vi "Data_PSD_267.vi"() -> ()   [LabVIEW 2020]
uses:
  <vilib>/Utility/error.llb/DialogType.ctl
  <vilib>/measure/maspectr.llb/Power Spectrum and PSD Export Mode.ctl
  <vilib>/Analysis/4window.llb/windowTd.ctl
  <vilib>/measure/maspectr.llb/FFT Power Spectrum and PSD for 1 Chan.vi
  <vilib>/Analysis/0measdsp.llb/Scaled Time Domain Window (DBL).vi
  <vilib>/sound2/lvsound2.llb/Sound File Info (path).vi
  <vilib>/sound2/lvsound2.llb/Sound File Read Open.vi
  <vilib>/sound2/lvsound2.llb/Sound File Read (DBL).vi
  <vilib>/Analysis/NI_AALPro.lvlib
  <vilib>/measure/NI_MAPro.lvlib
panel:
  in  "Stop":bool
  out "Data Cursor":T1
  in  "File Path":path
  out "Max Amplitude":dbl
  out "Frequency Peak":dbl
  out "Signal":waveform(dbl)(graph)
  out "PSD of Signal":cluster{"f0":dbl, "df":dbl, "magnitude":dbl[]}(graph)
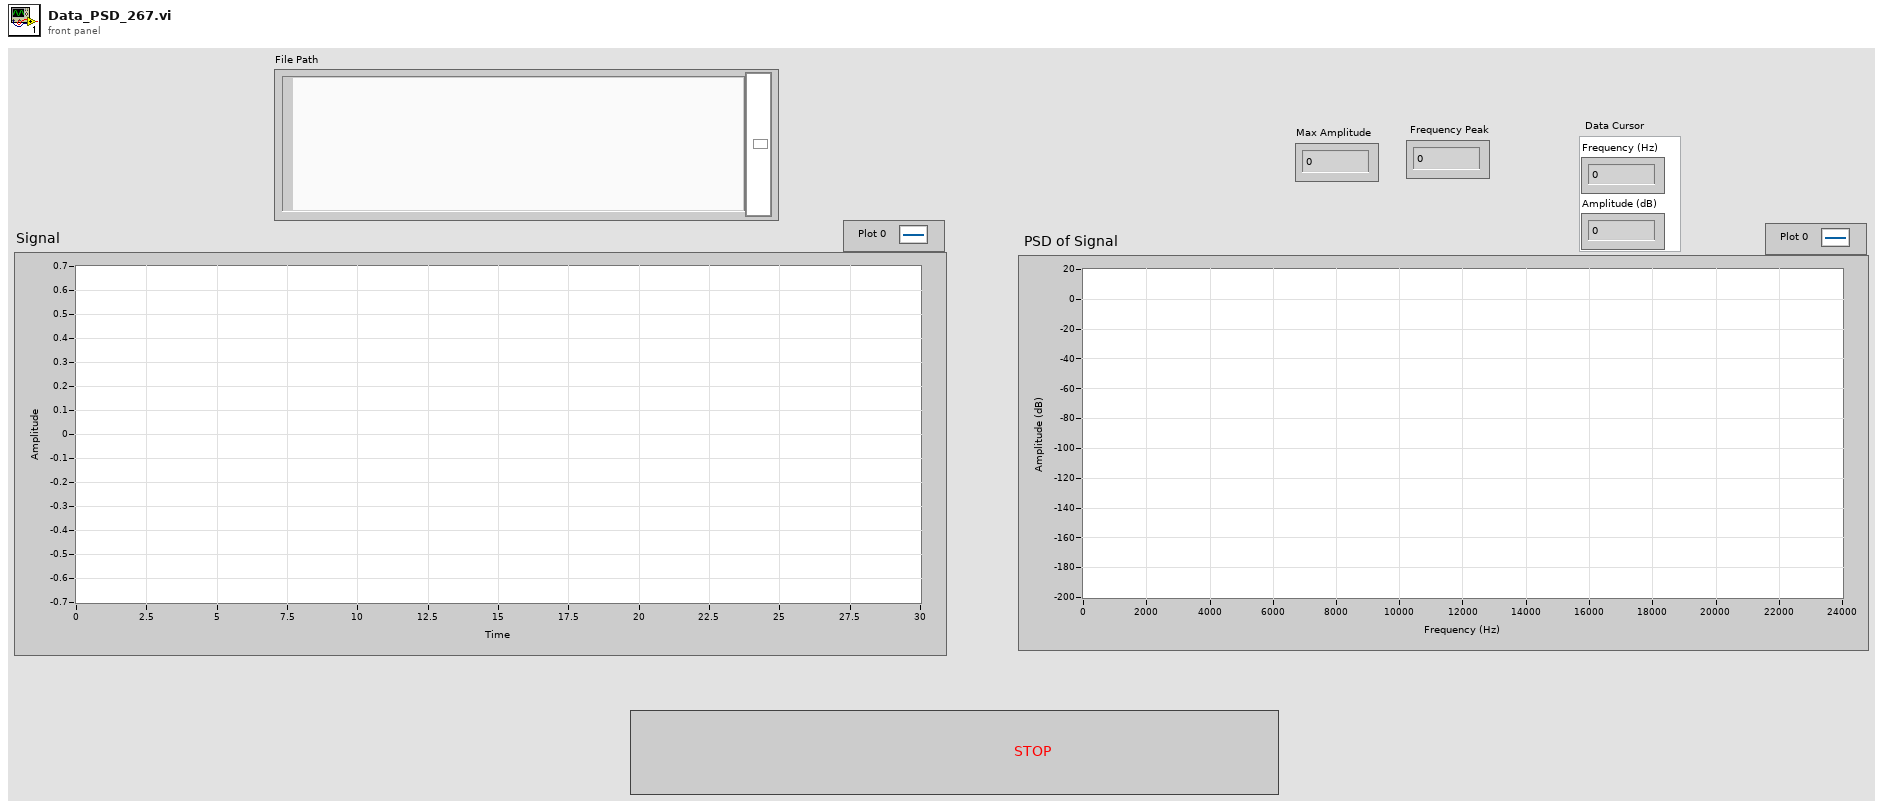
[diagram p1: front panel]
types:
  T1 = cluster{"Frequency (Hz)":dbl, "Amplitude (dB)":dbl}
  T2 = typedef "DialogType.ctl" = u16
  T3 = typedef "NI_AALPro.lvlib/windowTd.ctl" = u32
  T4 = typedef "NI_MAPro.lvlib/Power Spectrum and PSD Export Mode.ctl" = u16
  T5 = typedef "LVPointDoubleTypeDef.ctl" = cluster{"Cursor X":dbl, "Cursor Y":dbl}
  T6 = typedef "Sound File Refnum.ctl" = refnum<file>
  T7 = typedef "LVRangeTypeDef.ctl" = cluster{"Minimum":dbl, "Maximum":dbl, "Increment":dbl, "Minor Increment":dbl, "Start":dbl}
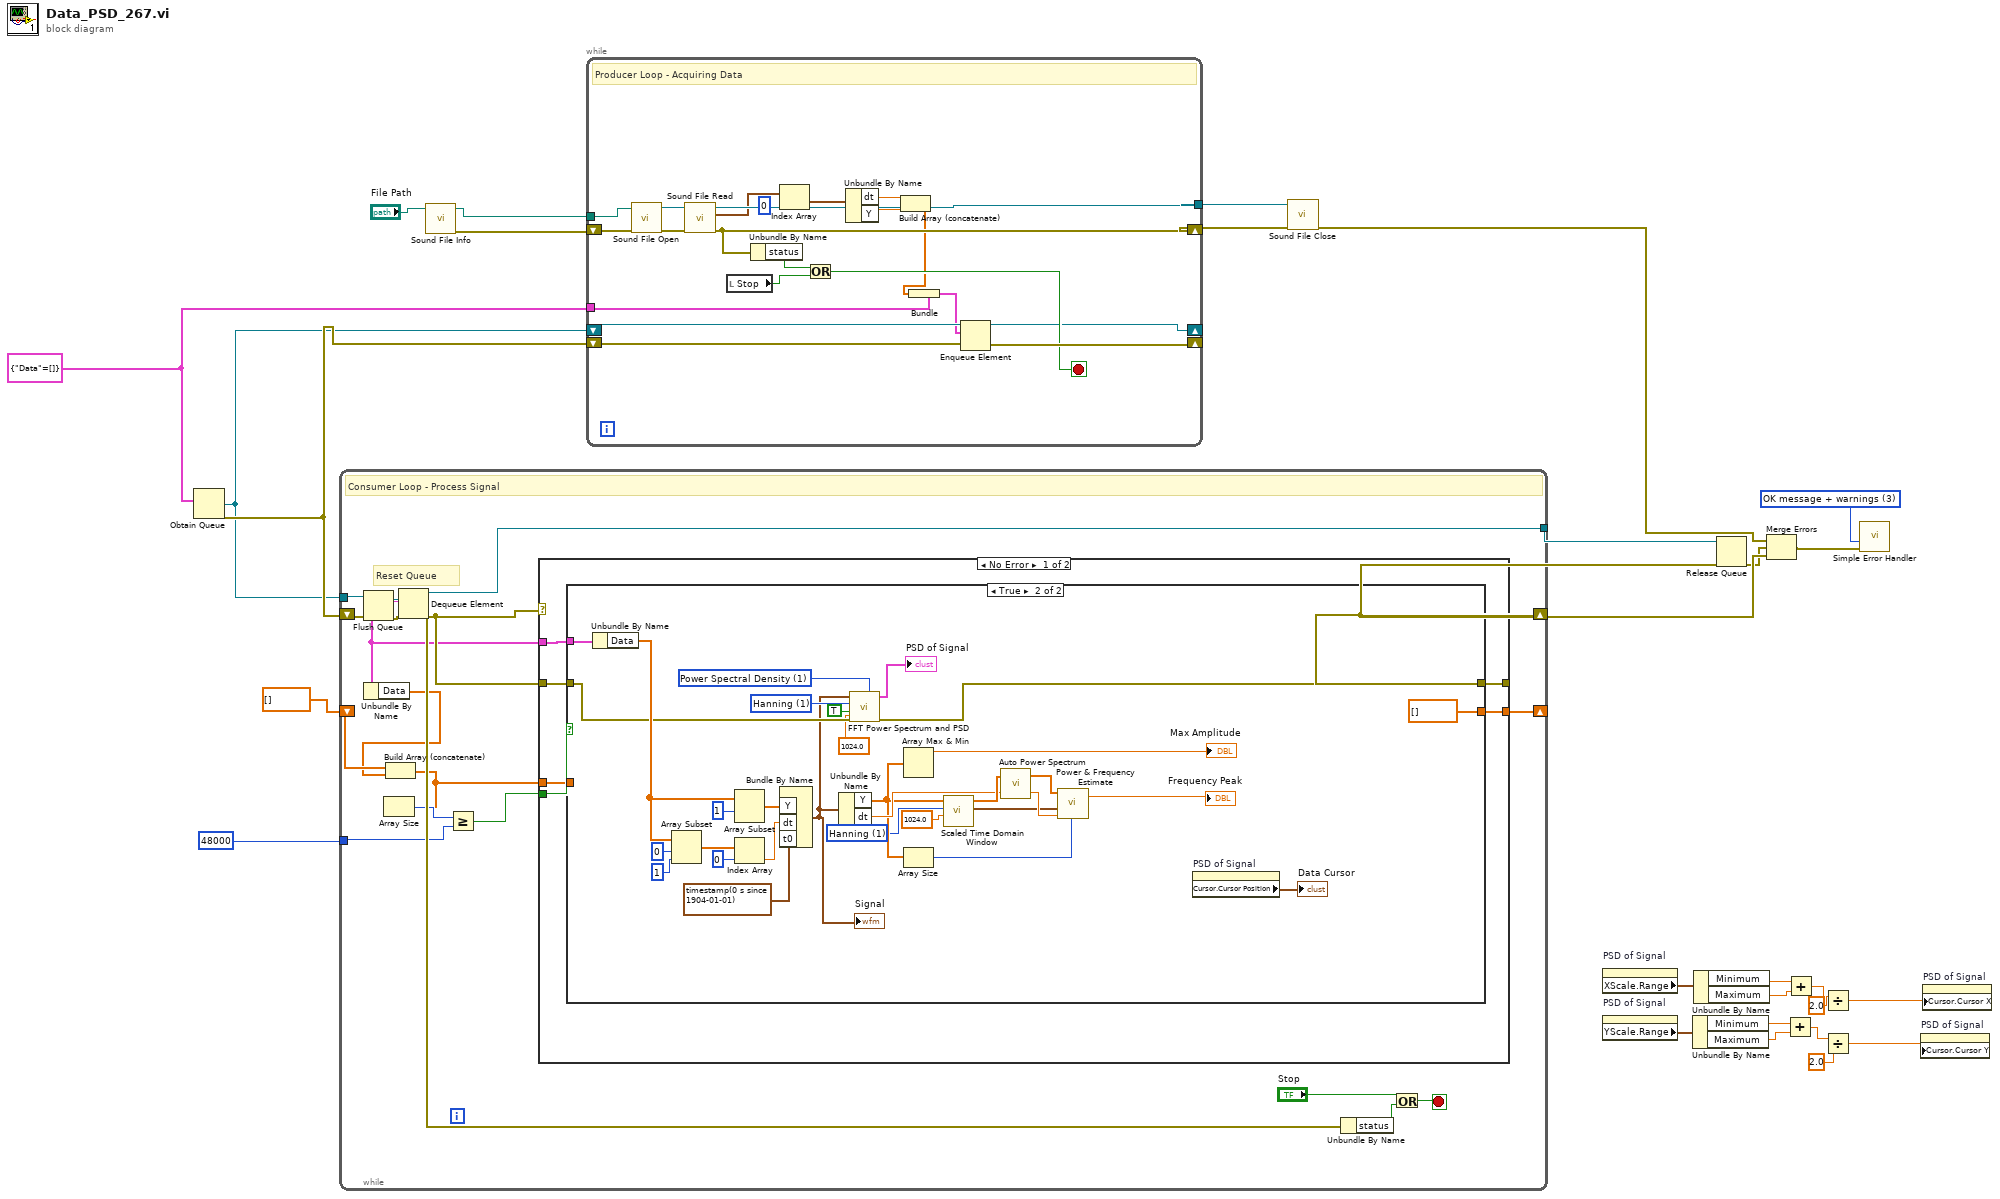
[diagram p0: block diagram]
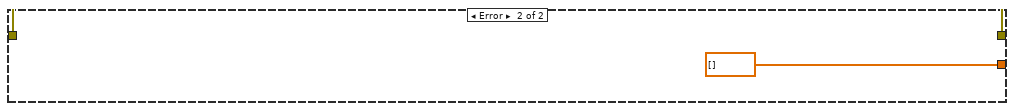
[diagram p3: hidden frame]
diagram:
  w16 = cluster{"Data":dbl[]} {"Data"=[]}
  w28 = T2 3 items=["no dialog", "OK message", "continue or stop message", "OK message + warnings", "continue/stop + warnings"] ("type of dialog (OK msg:1)")
  n1 = Obtain Queue(element data type=w16) -> (queue out=w17:refnum<queue>, error out=w18:errorcluster)  [unwired: 3 in, 2 out]
  n2 = while {
    tunnel: w17 -> [w43]
    shift-right: [w46] -> w25
    shift-left: w18 -> [w41]
    tunnel: [w39] -> w26
    tunnel: 48000 -> [w35]
    shift-right: [w31] -> _
    shift-left: dbl[] [] -> [w36]
    stop <- w44 stop-if-true
    # "Reset Queue"
    # "Consumer Loop - Process Signal"
    n3 = Flush Queue(queue=w43, error in (no error)=w41) -> (queue out=w42:refnum<queue>, error out=w40:errorcluster)  [unwired: 1 out]
    n4 = Dequeue Element(queue=w42, error in (no error)=w40) -> (queue out=w39:refnum<queue>, element=w37:cluster{"Data":dbl[]}, error out=w38:errorcluster)  [unwired: 2 out]
    n5 = Unbundle By Name(w37) -> ("Data"=w32:dbl[])
    n6 = Build Array (concatenate)(w36, w32) -> (w30:dbl[])
    n7 = Array Size(array=w30) -> (size(s)=w34:i32)
    n8 = Greater Or Equal?(x=w34, y=w35) -> (x >= y?=w33:bool)
    n9 = case shown="No Error" w38 {
      tunnel: w37 -> [w52 _]
      tunnel: [w47 w87] -> w46
      tunnel: w38 -> [w48 w87]
      tunnel: w33 -> [w51 _]
      tunnel: [w50 dbl[] []] -> w31
      tunnel: w30 -> [w49 _]
      frame No Error {
        n10 = case shown="True" w51 {
          tunnel: w52 -> [_ w67]
          tunnel: [w54 dbl[] []] -> w50
          tunnel: w49 -> [w54 _]
          tunnel: w48 -> [w53 w63]
          tunnel: [w53 w62] -> w47
          frame False {
          }
          frame True {
            w68 = T3 1 items=["Rectangle"=0, "Hanning"=1, "Hamming"=2, "Blackman-Harris"=3, "Exact Blackman"=4, "Blackman"=5, "Flat Top"=6, "4 Term B-Harris "=7, "7 Term B-Harris"=8, "Low Sidelobe"=9, "Blackman Nuttall"=11, "Triangle"=30, "Bartlett-Hanning"=31, "Bohman"=32, "Parzen"=33, "Welch"=34, "Kaiser"=60, "Dolph-Chebyshev"=61, "Gaussian"=62] ("window")
            w69 = T3 1 items=["Rectangle"=0, "Hanning"=1, "Hamming"=2, "Blackman-Harris"=3, "Exact Blackman"=4, "Blackman"=5, "Flat Top"=6, "4 Term B-Harris "=7, "7 Term B-Harris"=8, "Low Sidelobe"=9, "Blackman Nuttall"=11, "Triangle"=30, "Bartlett-Hanning"=31, "Bohman"=32, "Parzen"=33, "Welch"=34, "Kaiser"=60, "Dolph-Chebyshev"=61, "Gaussian"=62] ("window")
            w82 = T4 1 items=["Power Spectrum", "Power Spectral Density"] ("export mode")
            n11 = Unbundle By Name(w67) -> ("Data"=w66:dbl[])
            n12 = Array Subset(array=w66, index=0, length=1) -> (w78:dbl[])
            n13 = Array Subset(array=w66, index=1) -> (w79:dbl[])  [unwired: 1 in]
            n14 = Index Array(array=w78, index=0) -> (element=w76:dbl)
            n15 = Bundle By Name("Y"=w79, "dt"=w76, "t0"=timestamp(0 s since 1904-01-01)) -> (w58:waveform(dbl))  [unwired: 1 in]
            "Signal" <- w58
            n16 = Unbundle By Name(w58) -> ("Y"=w72:dbl[], "dt"=w81:dbl)
            n17 = call-poly <vilib>:"FFT Power Spectrum and PSD.vi"("window parameter"=1024.0, "export mode"=w82, "error in (no error)"=w63, "dB On (F)"=TRUE, "window"=w68, "time signal"=w58) -> ("error out"=w62:errorcluster, "Power Spectrum / PSD"=→"PSD of Signal":cluster{"f0":dbl, "df":dbl, "magnitude":dbl[]})  [unwired: 2 in, 2 out]
            n18 = Array Max & Min(array=w72) -> (max value=→"Max Amplitude":dbl)  [unwired: 3 out]
            n19 = Array Size(array=w72) -> (size(s)=w71:i32)
            n20 = call-poly <vilib>:"Scaled Time Domain Window.vi"("window parameter"=1024.0, "window"=w69, "X"=w72) -> ("window properties"=w70:cluster{"eq noise BW":dbl, "coherent gain":dbl}, "Windowed X"=w84:dbl[])  [unwired: 7 out]
            n21 = call <vilib>:"Auto Power Spectrum.vi"("dt"=w81, "Signal (V)"=w84) -> ("df"=w85:dbl, "Power Spectrum (V^2 rms)"=w73:dbl[])
            n22 = call <vilib>:"Power & Frequency Estimate.vi"("span"=w71, "df"=w85, "window constants"=w70, "Power Spectrum (V^2 rms)"=w73) -> ("est frequency peak"=→"Frequency Peak":dbl)  [unwired: 1 in, 2 out]
            n23 = property on="PSD of Signal" class="WFGraph (strict)"() -> ("Cursor.Cursor Position"=→"Data Cursor":T5)  [unwired: 2 in, 2 out]
          }
        }
      }
      frame Error {
      }
    }
    n24 = Unbundle By Name(w38) -> ("status"=w45:bool)
    n25 = Or(x="Stop", y=w45) -> (x .or. y?=w44:bool)
  }
  n26 = call-poly <vilib>:"Sound File Info.vi"("path"="File Path") -> ("error out"=w21:errorcluster, "path out"=w22:path)  [unwired: 7 in, 2 out]
  n27 = while {
    shift-right: [w107] -> _
    shift-left: w18 -> [w108]
    shift-right: [w96] -> w19
    shift-left: w21 -> [w102]
    tunnel: w22 -> [w104]
    tunnel: [w100] -> w20
    shift-right: [w90] -> _
    shift-left: w17 -> [w92]
    tunnel: w16 -> [w89]
    stop <- w105 stop-if-true
    # "Producer Loop - Acquiring Data"
    n28 = call-poly <vilib>:"Sound File Open.vi"("error in (no error)"=w102, "path"=w104) -> ("error out"=w101:errorcluster, "sound file refnum"=w103:T6)  [unwired: 8 in]
    n29 = call-poly <vilib>:"Sound File Read.vi"("error in (no error)"=w101, "sound file refnum"=w103) -> ("error out"=w96:errorcluster, "data"=w99:waveform(dbl)[], "sound file refnum out"=w100:T6)  [unwired: 5 in, 2 out]
    n30 = local read "Stop"() -> (w88:bool)
    n31 = Unbundle By Name(w96) -> ("status"=w106:bool)
    n32 = Index Array(array=w99, index=0) -> (element=w97:waveform(dbl))
    n33 = Or(x=w106, y=w88) -> (x .or. y?=w105:bool)
    n34 = Unbundle By Name(w97) -> ("dt"=w95:dbl, "Y"=w94:dbl[])
    n35 = Build Array (concatenate)(w95, w94) -> (w93:dbl[])
    n36 = Bundle(cluster=w89, "Data"=w93) -> (w91:cluster{"Data":dbl[]})
    n37 = Enqueue Element(queue=w92, element=w91, error in (no error)=w108) -> (queue out=w90:refnum<queue>, error out=w107:errorcluster)  [unwired: 2 out]
  }
  n38 = call <vilib>:"Sound File Close.vi"("error in (no error)"=w19, "sound file refnum"=w20) -> ("error out"=w15:errorcluster)  [unwired: 9 in]
  n39 = property on="PSD of Signal" class="WFGraph (strict)"() -> ("XScale.Range"=w12:T7)  [unwired: 2 in, 2 out]
  n40 = property on="PSD of Signal" class="WFGraph (strict)"() -> ("YScale.Range"=w11:T7)  [unwired: 2 in, 2 out]
  n41 = Unbundle By Name(w11) -> ("Minimum"=w4:dbl, "Maximum"=w3:dbl)
  n42 = Unbundle By Name(w12) -> ("Minimum"=w10:dbl, "Maximum"=w9:dbl)
  n43 = Release Queue(queue=w26, error in (no error)=w25) -> (error out=w24:errorcluster)  [unwired: 1 in, 2 out]
  n44 = Merge Errors(w15, w24, w25) -> (w27:errorcluster)
  n45 = Add(x=w4, y=w3) -> (x+y=w6:dbl)
  n46 = Add(x=w10, y=w9) -> (x+y=w7:dbl)
  n47 = Divide(x=2.0 ("y"), y=w7) -> (x/y=w1:dbl)
  n48 = Divide(x=w6, y=2.0) -> (x/y=w2:dbl)
  n49 = call <vilib>:"Simple Error Handler.vi"("type of dialog (OK msg:1)"=w28, "error in (no error)"=w27) -> ()  [unwired: 8 out]
  n50 = property on="PSD of Signal" class="WFGraph (strict)"("Cursor.Cursor Y"=w2) -> ()  [unwired: 2 in, 2 out]
  n51 = property on="PSD of Signal" class="WFGraph (strict)"("Cursor.Cursor X"=w1) -> ()  [unwired: 2 in, 2 out]
